vi "STS Calculator_2014_05_29_PD.vi"(8 "NumPts":i32=3, 10 "Saturation Id":dbl[](array[numeric]), 11 "Vg Column":dbl[](array[numeric])) -> (0 "STS Index":dbl, 2 "XY Graph":cluster{dbl[], dbl[]}[](graph), 3 "Sub Threshold Swing":dbl, 5 "Used Points":cluster{"Vg Used":dbl[], "Id Used":dbl[]})   [LabVIEW 2012]
uses:
  <vilib>/Analysis/NI_AALPro.lvlib
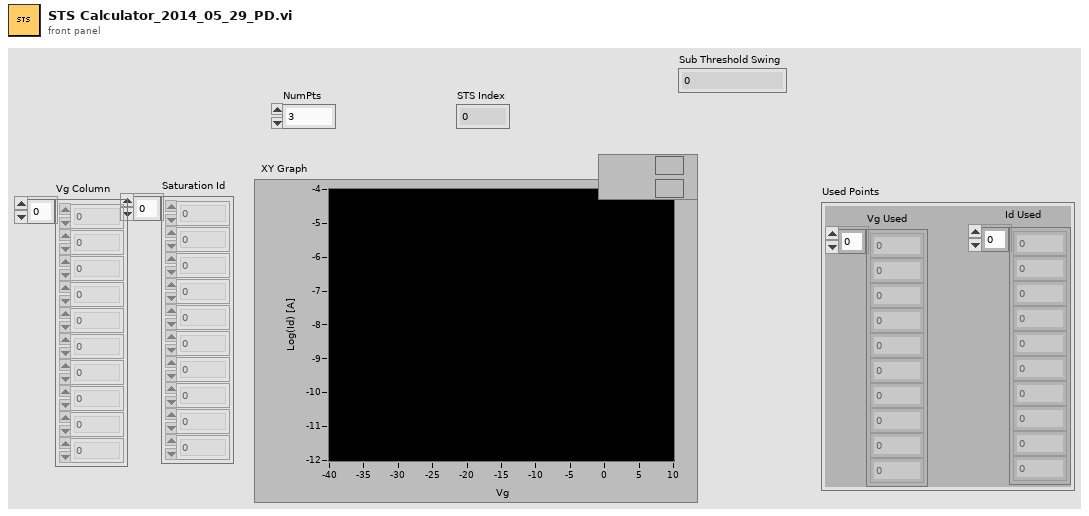
[diagram p1: front panel]
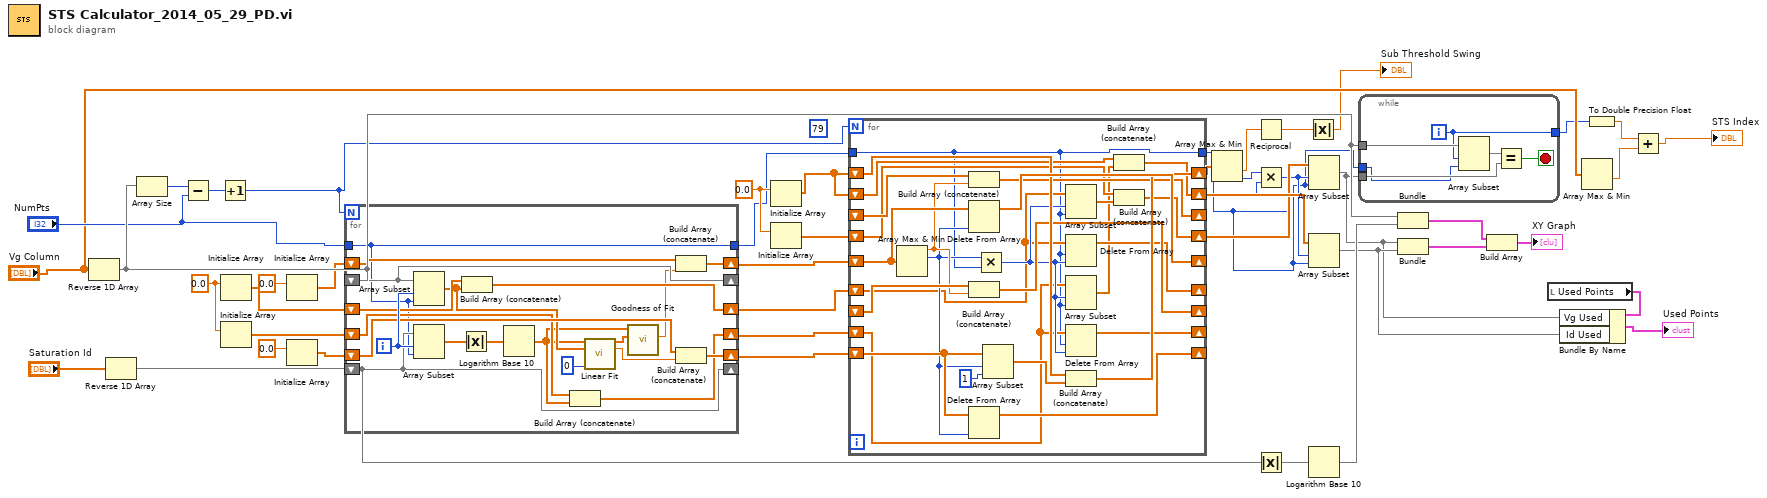
[diagram p0: block diagram]
diagram:
  w24 = 0.0
  w30 = 0.0
  (unwired) 79
  n1 = Reverse 1D Array(array="Vg Column") -> (reversed array=w41:dbl[])
  n2 = Reverse 1D Array(array="Saturation Id") -> (reversed array=w12:dbl[])
  n3 = Array Size(array=w41) -> (size(s)=w40:i32)
  n4 = Subtract(x=w40, y="NumPts") -> (x-y=w17:i32)
  n5 = Increment(x=w17) -> (x+1=w1:i32)
  n6 = Initialize Array(w30) -> (w28:dbl[])  [unwired: 1 in]
  n7 = Initialize Array(w30) -> (w29:dbl[])  [unwired: 1 in]
  n8 = Initialize Array(0.0) -> (w38:dbl[])  [unwired: 1 in]
  n9 = Initialize Array(0.0) -> (w39:dbl[])  [unwired: 1 in]
  n10 = for {
    N: w1 -> [_]
    shift-right: [w53] -> _
    shift-left: w41 -> [w53]
    shift-right: [w59] -> _
    shift-left: w12 -> [w59]
    shift-right: [w63] -> w35
    shift-left: w39 -> [w62]
    shift-right: [w61] -> w33
    shift-left: w38 -> [w60]
    tunnel: "NumPts" -> [w46]
    shift-right: [w56] -> w27
    shift-left: w29 -> [w57]
    shift-right: [w54] -> w26
    shift-left: w28 -> [w55]
    tunnel: [w46] -> w8
    i -> [w65]
    n11 = Array Subset(array=w53, index=w65, length=w46) -> (w52:dbl[])
    n12 = Array Subset(array=w59, index=w65, length=w46) -> (w47:dbl[])
    n13 = Absolute Value(x=w47) -> (abs(x)=w48:dbl[])
    n14 = Build Array (concatenate)(w55, w52) -> (w54:dbl[])
    n15 = Logarithm Base 10(1:w48) -> (0:w49:dbl[])
    n16 = Build Array (concatenate)(w57, w49) -> (w56:dbl[])
    n17 = call <vilib>:"Linear Fit.vi"("Y"=w49, "X"=w52, "method"=0) -> ("Best Linear Fit"=w51:dbl[], "slope"=w64:dbl)  [unwired: 8 in, 3 out]
    n18 = call <vilib>:"Goodness of Fit.vi"("Best Fit"=w51, "Y"=w49) -> ("R-square"=w50:dbl)  [unwired: 6 in, 3 out]
    n19 = Build Array (concatenate)(w60, w50) -> (w61:dbl[])
    n20 = Build Array (concatenate)(w62, w64) -> (w63:dbl[])
  }
  n21 = Initialize Array(w24) -> (w20:dbl[])  [unwired: 1 in]
  n22 = Initialize Array(w24) -> (w25:dbl[])  [unwired: 1 in]
  n23 = for {
    N: w1 -> [_]
    shift-right: [w90] -> _
    shift-left: w33 -> [w91]
    shift-right: [w71] -> _
    shift-left: w35 -> [w72]
    shift-right: [w87] -> w34
    shift-left: w20 -> [w86]
    shift-right: [w85] -> _
    shift-left: _ -> [w84]
    shift-right: [w83] -> _
    shift-left: _ -> [w82]
    shift-right: [w81] -> _
    shift-left: w27 -> [w68]
    shift-right: [w79] -> _
    shift-left: w26 -> [w67]
    tunnel: w8 -> [w66]
    shift-right: [w78] -> w23
    shift-left: w20 -> [w77]
    shift-right: [w76] -> w22
    shift-left: w25 -> [w75]
    tunnel: [w66] -> w7
    n24 = Array Max & Min(array=w91) -> (max value=w70:dbl, max index (indices)=w69:i32)  [unwired: 2 out]
    n25 = Build Array (concatenate)(w82, w70) -> (w83:dbl[])
    n26 = Delete From Array(array=w91, index=w69) -> (array with subset deleted=w90:dbl[])  [unwired: 1 in, 1 out]
    n27 = Build Array (concatenate)(w84, w70) -> (w85:dbl[])
    n28 = Delete From Array(array=w72, index=w69) -> (array with subset deleted=w71:dbl[])  [unwired: 1 in, 1 out]
    n29 = Multiply(x=w69, y=w66) -> (x*y=w80:i32)
    n30 = Array Subset(array=w72, index=w69, length=1) -> (w88:dbl[])
    n31 = Array Subset(array=w67, index=w80, length=w66) -> (w74:dbl[])
    n32 = Delete From Array(array=w67, length=w66, index=w80) -> (array with subset deleted=w79:dbl[])  [unwired: 1 out]
    n33 = Array Subset(array=w68, index=w80, length=w66) -> (w73:dbl[])
    n34 = Delete From Array(array=w68, length=w66, index=w80) -> (array with subset deleted=w81:dbl[])  [unwired: 1 out]
    n35 = Build Array (concatenate)(w86, w88) -> (w87:dbl[])
    n36 = Build Array (concatenate)(w77, w73) -> (w78:dbl[])
    n37 = Build Array (concatenate)(w75, w74) -> (w76:dbl[])
  }
  n38 = Array Max & Min(array=w34) -> (min value=w44:dbl, min index (indices)=w21:i32)  [unwired: 2 out]
  n39 = Reciprocal(x=w44) -> (1/x=w45:dbl)
  n40 = Multiply(x=w21, y=w7) -> (x*y=w19:i32)
  n41 = Absolute Value(x=w12) -> (abs(x)=w43:dbl[])
  n42 = Absolute Value(x=w45) -> (abs(x)=→"Sub Threshold Swing":dbl)
  n43 = Array Subset(array=w22, index=w19, length=w7) -> (w14:dbl[])
  n44 = Array Subset(array=w23, index=w19, length=w7) -> (w15:dbl[])
  n45 = Logarithm Base 10(1:w43) -> (0:w42:dbl[])
  n46 = while {
    tunnel: w41 -> [w96]
    tunnel: w14 -> [w95]
    tunnel: [w93] -> w3
    tunnel: w7 -> [w92]
    i -> [w93]
    stop <- w97 stop-if-true
    n47 = Array Subset(array=w96, index=w93, length=w92) -> (w94:dbl[])
    n48 = Equal?(x=w94, y=w95) -> (x = y?=w97:bool)
  }
  n49 = Bundle(w41, w42) -> (w31:cluster{dbl[], dbl[]})  [unwired: 1 in]
  n50 = Bundle(w14, w15) -> (w18:cluster{dbl[], dbl[]})  [unwired: 1 in]
  n51 = Build Array(w31, w18) -> (→"XY Graph":cluster{dbl[], dbl[]}[])
  n52 = local read "Used Points"() -> (w16:cluster{"Vg Used":dbl[], "Id Used":dbl[]})
  n53 = Bundle By Name(cluster=w16, "Vg Used"=w14, "Id Used"=w15) -> (→"Used Points":cluster{"Vg Used":dbl[], "Id Used":dbl[]})
  n54 = Array Max & Min(array="Vg Column") -> (min value=w11:dbl)  [unwired: 3 out]
  n55 = To Double Precision Float(number=w3) -> (double precision float=w2:dbl)
  n56 = Add(x=w2, y=w11) -> (x+y=→"STS Index":dbl)
